vi "Setup Test Runner.vi"(8 "error in (no error)":errorcluster, 9 "Report Path":path, 10 "Directory to search":path) -> (0 "error out":errorcluster, 3 "Test Runner out":refnum<class "Test Runner.lvclass">)   [LabVIEW 2013, in "Caraya.lvlib" / "Test Runner.lvclass"]
uses:
  Test Runner.lvclass
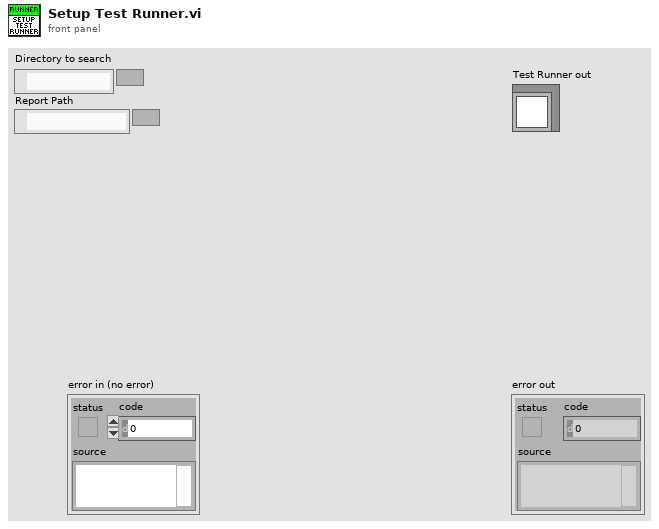
[diagram p1: front panel]
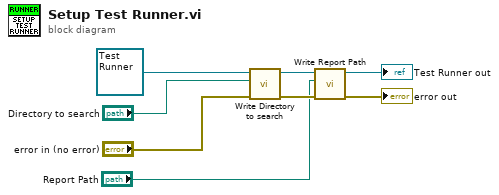
[diagram p0: block diagram]
diagram:
  n1 = call-dynamic "Write Directory to search.vi"("error in (no error)"="error in (no error)", "Directory to search"="Directory to search", "Test Runner in"=refnum<class "Test Runner.lvclass"> refnum) -> ("error out"=w7:errorcluster, "Test Runner out"=w8:refnum<class "Test Runner.lvclass">)  [unwired: 7 in]
  n2 = call-dynamic "Write Report Path.vi"("error in (no error)"=w7, "Report Path"="Report Path", "Test Runner in"=w8) -> ("error out"=→"error out":errorcluster, "Test Runner out"=→"Test Runner out":refnum<class "Test Runner.lvclass">)  [unwired: 7 in]
